vi "emitters 2 PDWs.vi"(8 "error in (no error)":errorcluster, 9 "random startinig phase":bool, 10 "emmiter":T3[](array[typedef]) {"t end" format="%#_3p"; "t start" format="%#_3p"; "DOA" format="%#_3p"}, 11 "device_type in":refnum<class "device_type.lvclass">) -> (0 "error out":errorcluster, 2 "sorted PDWs":T1[](array[typedef]), 3 "device_type out":refnum<class "device_type.lvclass">)   [LabVIEW 2021, in "device_type.lvclass"]
uses:
  device_type.lvclass
  pulse_tx_vis/CTL/emitter params.ctl
  pulse_tx_vis/CTL/mode_type.ctl
  pulse_tx_vis/CTL/PDW_lv2.ctl
  device_type.lvclass/device_type.ctl
  2197b3eb-2394-420c-90e9-03a4284ab46f.vi
  <vilib>/Comparison/Less/Less Functor/Less Functor.lvclass
panel:
  out "may saturate":bool
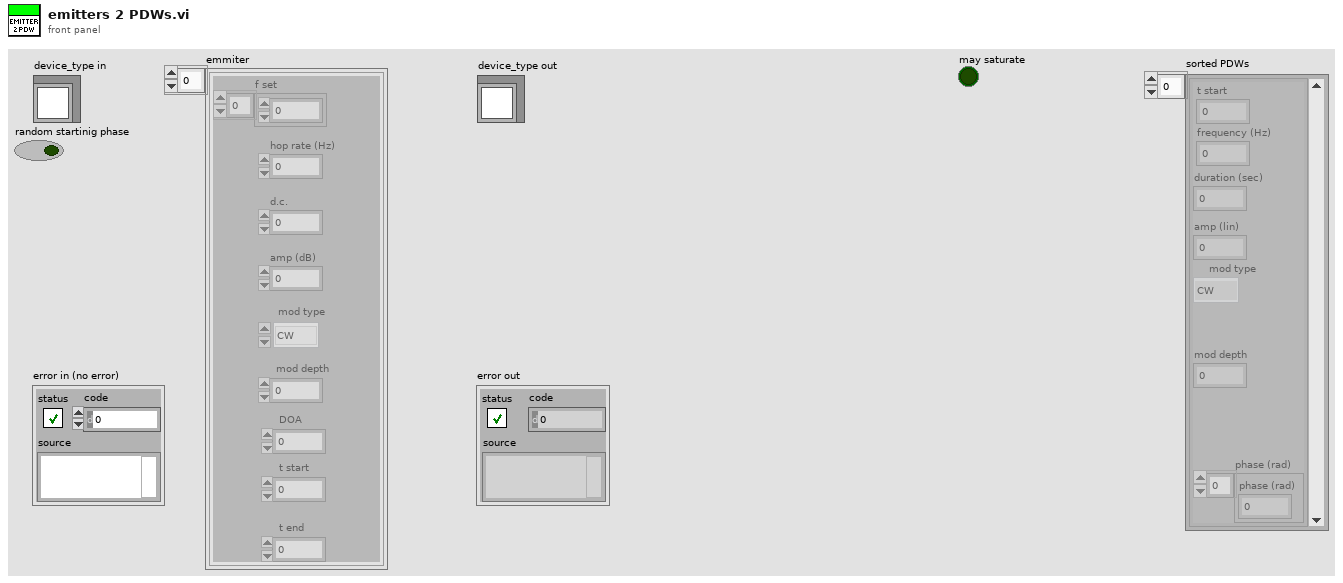
[diagram p1: front panel]
types:
  T1 = typedef "PDW_lv2.ctl" = cluster{"t start":dbl, "frequency (Hz)":dbl, "duration (sec)":dbl, "amp (lin)":dbl, "mod type":T2, "mod depth":dbl, "phase (rad)":dbl[]}
  T2 = typedef "mode_type.ctl" = enum8{"CW", "from memory 1", "NC - cw", "LFM", "BPSK", "QPSK"}
  T3 = typedef "emitter params.ctl" = cluster{"f set":dbl[], "hop rate (Hz)":dbl, "d.c.":dbl, "amp (dB)":dbl, "mod type":T2, "mod depth":dbl, "DOA":dbl, "t start":dbl, "t end":dbl}
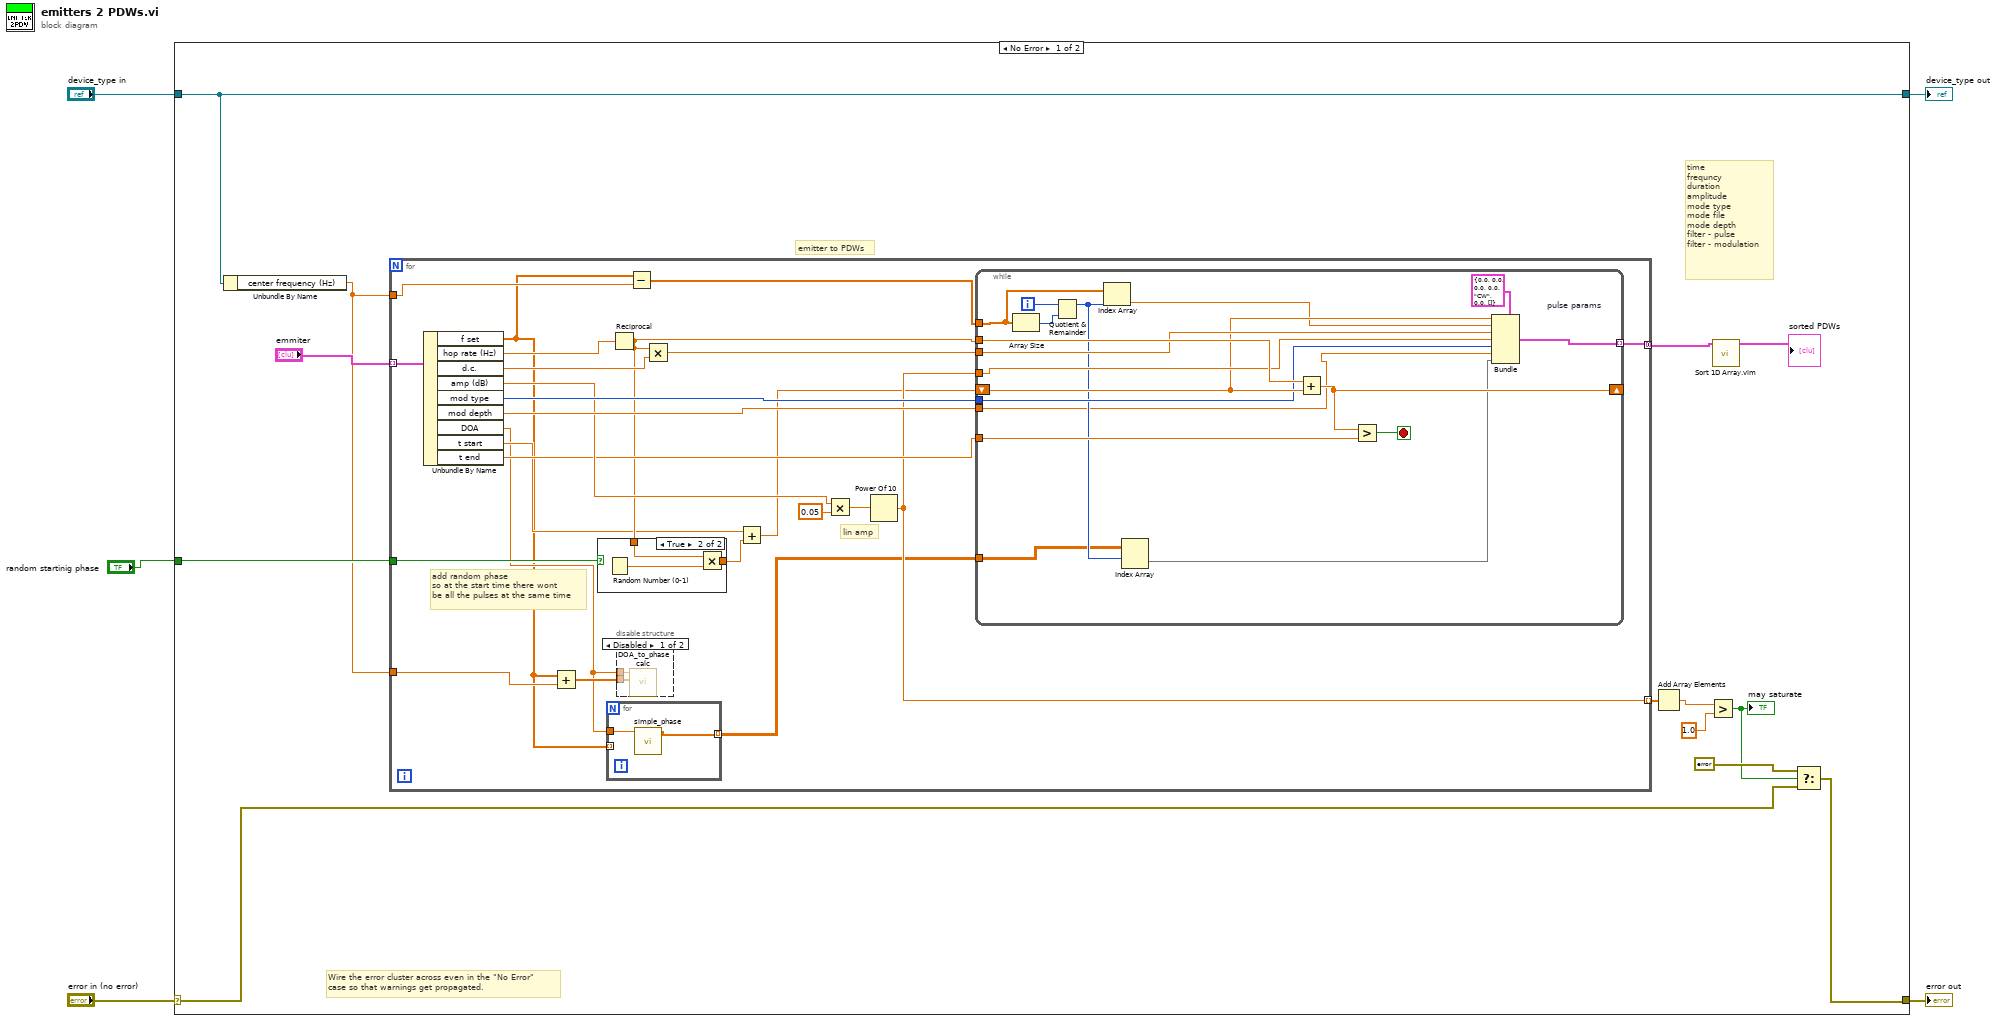
[diagram p0: block diagram]
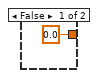
[diagram p3: hidden frame]
diagram:
  n1 = case shown="No Error" "error in (no error)" {
    selector: "error in (no error)" -> [w9 w70]
    tunnel: [w8 w70] -> w4
    tunnel: [w10 w69] -> w2
    tunnel: "device_type in" -> [w10 w69]
    tunnel: "random startinig phase" -> [w7 _]
    frame No Error {
      # "time\nfrequncy\nduration\namplitude\nmode type\nmode file\nmode depth\nfilter - pulse\nfilter - modulation"
      # "emitter to PDWs"
      # "Wire the error cluster across even in the \"No Error\"\ncase so that warnings get propagated."
      n2 = Unbundle By Name(w10) -> ("center frequency (Hz)"=w6:dbl)
      n3 = for {
        tunnel: "emmiter" -> [w42] mode=indexing
        tunnel: [w39] -> w18 mode=concatenating
        tunnel: w6 -> [w30]
        tunnel: [w28] -> w16 mode=indexing
        tunnel: w7 -> [w24]
        tunnel: w6 -> [w23]
        # "add random phase \nso at the start time there wont\nbe all the pulses at the same time"
        # "lin amp"
        n4 = Unbundle By Name(w42) -> ("f set"=w20:dbl[], "hop rate (Hz)"=w36:dbl, "d.c."=w41:dbl, "amp (dB)"=w33:dbl, "mod type"=w38:T2, "mod depth"=w37:dbl, "DOA"=w21:dbl, "t start"=w27:dbl, "t end"=w32:dbl)
        n5 = Add(x=w20, y=w30) -> (x+y=w29:dbl[])
        n6 = for {
          tunnel: w21 -> [w46]
          tunnel: w20 -> [_] mode=indexing
          tunnel: [w45] -> w19 mode=indexing
          n7 = call "simple_phase.vi"("DOA"=w46) -> ("simple phase"=w45:dbl[])  [unwired: 10 in]
        }
        n8 = Reciprocal(x=w36) -> (1/x=w31:dbl)
        n9 = case shown="True" w24 {
          tunnel: w31 -> [_ w50]
          tunnel: [0.0 w48] -> w26
          frame False {
          }
          frame True {
            n10 = Random Number (0-1)() -> (number: 0 to 1=w49:dbl)
            n11 = Multiply(x=w50, y=w49) -> (x*y=w48:dbl)
          }
        }
        n12 = disable-structure shown="Disabled" {
          disable-tunnel: w29 -> [w44 _]
          disable-tunnel: w21 -> [w43 _]
          frame Disabled {
            n13 = call "DOA_to_phase calc.vi"("f set (Hz)"=w44, "DOA (deg)"=w43) -> ()  [unwired: 9 in, 1 out]
          }
          frame Enabled {
          }
        }
        n14 = Subtract(x=w20, y=w23) -> (x-y=w22:dbl[])
        n15 = Multiply(x=w31, y=w41) -> (x*y=w40:dbl)
        n16 = Add(x=w27, y=w26) -> (x+y=w25:dbl)
        n17 = Multiply(x=w33, y=0.05) -> (x*y=w34:dbl)
        n18 = Power Of 10(x=w34) -> (10^x=w28:dbl)
        n19 = while {
          tunnel: w22 -> [w66]
          shift-right: [w63] -> _
          shift-left: w25 -> [w58]
          tunnel: w31 -> [w65]
          tunnel: w32 -> [w64]
          tunnel: w40 -> [w61]
          tunnel: w28 -> [w60]
          tunnel: [w59] -> w39 mode=indexing
          tunnel: w38 -> [w56]
          tunnel: w37 -> [w51]
          tunnel: w19 -> [w54]
          i -> [w68]
          stop <- w62 stop-if-true
          n20 = Array Size(array=w66) -> (size(s)=w67:i32)
          n21 = Quotient & Remainder(x=w68, y=w67) -> (x-y*floor(x/y)=w55:i32)  [unwired: 1 out]
          n22 = Index Array(array=w66, index=w55) -> (element=w57:dbl)
          n23 = Index Array(array=w54, index (row)=w55) -> (element=w52:dbl[])  [unwired: 1 in]
          n24 = Add(x=w65, y=w58) -> (x+y=w63:dbl)
          n25 = Greater?(x=w63, y=w64) -> (0:w62:bool)
          n26 = Bundle "pulse params"(cluster=T1 {"t start"=0.0, "frequency (Hz)"=0.0, "duration (sec)"=0.0, "amp (lin)"=0.0, "mod type"=enum."CW", "mod depth"=0.0, "phase (rad)"=[]} ("Cluster"), "t start"=w58, "frequency (Hz)"=w57, "duration (sec)"=w61, "amp (lin)"=w60, "mod type"=w56, "mod depth"=w51, "phase (rad)"=w52) -> (w59:T1)
        }
      }
      n27 = Add Array Elements(numeric array=w16) -> (sum=w15:dbl)
      n28 = Greater?(x=w15, y=1.0) -> (0:w12:bool)
      "may saturate" <- w12
      n29 = call "Sort 1D Array.vim"("unsorted array"=w18) -> ("sorted array"=→"sorted PDWs":T1[])  [unwired: 10 in]
      n30 = Select(t=errorcluster {"status"=FALSE, "code"=5432, "source"="the total amp of all the emmiters are higher then 1, if thay transmit togeder the output will saturate"} ("error out"), s=w12, f=w9) -> (s? t:f=w8:errorcluster)
    }
    frame Error {
    }
  }
  "error out" <- w4
  "device_type out" <- w2
